vi "PM100D_SensIDNFlag.vi"(2 "String":string) -> (0 "Wave?":bool, 1 "Resp?":bool, 3 "Ener?":bool, 4 "Flag":bool[](array[boolean]), 5 "Tau?":bool, 6 "Temp?":bool, 7 "Pow?":bool)   [LabVIEW 2014]
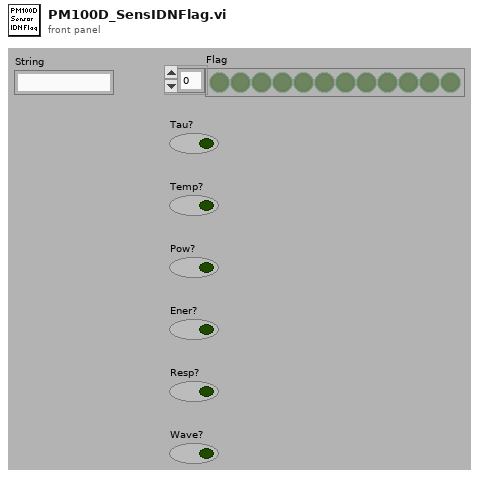
[diagram p1: front panel]
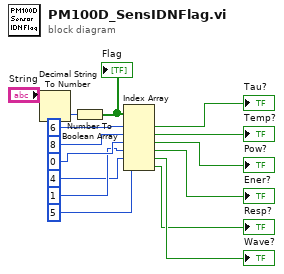
[diagram p0: block diagram]
diagram:
  n1 = Decimal String To Number(string="String") -> (number=w14:i32)  [unwired: 2 in, 1 out]
  n2 = Number To Boolean Array(number=w14) -> (Boolean array=w13:bool[])
  "Flag" <- w13
  n3 = Index Array(array=w13, index #1=6 ("index"), index #2=8 ("index"), index #3=0 ("index"), index #4=1 ("index"), index #5=4 ("index"), index #6=5 ("index")) -> (element #1=→"Tau?":bool, element #2=→"Temp?":bool, element #3=→"Pow?":bool, element #4=→"Ener?":bool, element #5=→"Wave?":bool, element #6=→"Resp?":bool)
